vi "Voronoi_Bounary Edges.vi"(8 "Centers":dbl[][](array[numeric]), 9 "Triangles":i32[][](array[numeric]), 10 "Y":dbl[](array[numeric]), 11 "X":dbl[](array[numeric])) -> (2 "Edge Y":dbl[][](array[numeric]), 3 "Edge X":dbl[][](array[numeric]))   [LabVIEW 2017, in "NI_AAL_Geometry.lvlib"]
uses:
  <vilib>/Analysis/NI_AAL_Geometry.lvlib
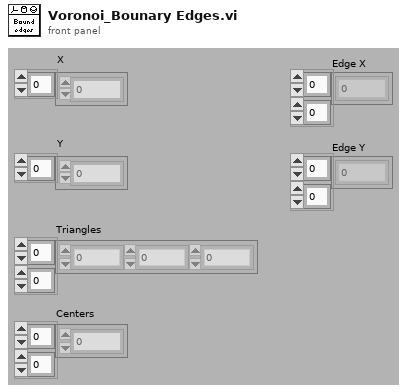
[diagram p1: front panel]
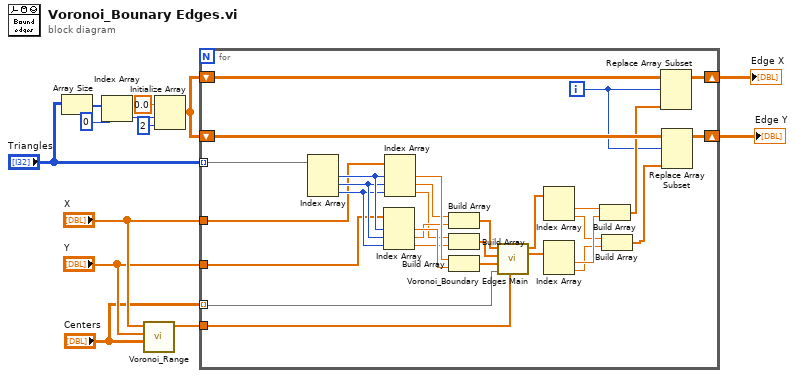
[diagram p0: block diagram]
diagram:
  n1 = Array Size(array="Triangles") -> (size(s)=w12:i32[])
  n2 = Index Array(array=w12, index=0) -> (element=w10:i32)
  n3 = call <vilib>:"Voronoi_Range.vi"("Centers"="Centers", "Y"="Y", "X"="X") -> ("Range"=w2:dbl[])  [unwired: 8 in]
  n4 = Initialize Array(0.0 ("element"), w10, 2 ("dimension size")) -> (w7:dbl[][])
  n5 = for {
    tunnel: "Triangles" -> [w25] mode=indexing
    tunnel: "X" -> [w24]
    tunnel: "Y" -> [w23]
    shift-right: [w19] -> w6
    shift-left: w7 -> [w20]
    shift-right: [w14] -> w5
    shift-left: w7 -> [w18]
    tunnel: w2 -> [w22]
    tunnel: "Centers" -> [w21] mode=indexing
    i -> [w15]
    n6 = Index Array(array=w25) -> (element #1=w36:i32, element #2=w35:i32, element #3=w34:i32)  [unwired: 3 in]
    n7 = Index Array(array=w23, index #1=w36, index #2=w35, index #3=w34) -> (element #1=w32:dbl, element #2=w30:dbl, element #3=w28:dbl)
    n8 = Index Array(array=w24, index #1=w36, index #2=w35, index #3=w34) -> (element #1=w33:dbl, element #2=w31:dbl, element #3=w29:dbl)
    n9 = Build Array(w31, w30) -> (w26:dbl[])
    n10 = Build Array(w29, w28) -> (w27:dbl[])
    n11 = Build Array(w33, w32) -> (w43:dbl[])
    n12 = call <vilib>:"Voronoi_Boundary Edges Main.vi"("Range"=w22, "Center"=w21, "P 3"=w43, "P 2"=w27, "P 1"=w26) -> ("End"=w38:dbl[], "Start"=w37:dbl[])  [unwired: 5 in]
    n13 = Index Array(array=w37) -> (element #1=w42:dbl, element #2=w40:dbl)  [unwired: 2 in]
    n14 = Index Array(array=w38) -> (element #1=w41:dbl, element #2=w39:dbl)  [unwired: 2 in]
    n15 = Build Array(w42, w41) -> (w17:dbl[])
    n16 = Build Array(w40, w39) -> (w16:dbl[])
    n17 = Replace Array Subset(array=w20, new element=w17, index (row)=w15) -> (w19:dbl[][])  [unwired: 1 in]
    n18 = Replace Array Subset(array=w18, new element=w16, index (row)=w15) -> (w14:dbl[][])  [unwired: 1 in]
  }
  "Edge X" <- w6
  "Edge Y" <- w5
